vi "Get Number AD Channels.vi"(11 "channels":i32) -> (2 "function return":u32, 3 "channels out":i32)   [LabVIEW 2018, in "AndorSDK.lvlib"]
doc: "EXPNETTYPE unsigned int WINAPI GetNumberADChannels(int * channels);"
uses:
  AndorSDK.lvlib
  ATMCD32D.dll
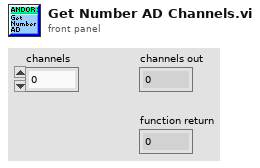
[diagram p1: front panel]
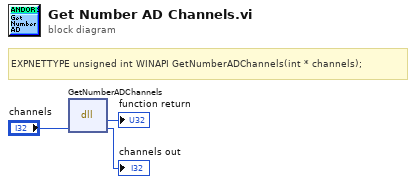
[diagram p0: block diagram]
diagram:
  # "EXPNETTYPE unsigned int WINAPI GetNumberADChannels(int * channels);"
  n1 = dll-call lib="PTH2babs E\nPersönliches02 - Arbeit03-HiwijobsLabviewCodelibANDOR\tAndor SDK\nATMCD32D.*" fn="GetNumberADChannels"("channels"="channels") -> (→"function return":u32, "channels"=→"channels out":i32)  [unwired: 3 in, 2 out]
